vi "Plot_Rectangle.vi"(3 "Mode":T5=enum."Run VI", 5 "Traverse line In":T2={"Start X"=-1250.0, "Start Y"=-250.0, "Start Z"=180.0, "End X"=0.0, "End Y"=0.0, "End Z"=0.0, "No. of pts."=6, "Spacing"=enum."Linear", "Filename"=path "C:/Enflo_Data_Local/2015/EnFlo_Tunnel/Paul_Hayden/Calibrations/Cal_06-2015/Datum_Block_1.xls", "Tunnel Speed"=0.0, "Averaging time (min)"=0.01, "Extra Commands"="", "Carrier_1 Q (l/min)"=nan, "Carrier_2 Q (l/min)"=nan, "Trace Gas Concentration (%)"=nan, "Specific Arguments"="Datum_Image_Calibration.vi  ", "Comments"="", "Row No"=0, "Row Type Selector"=enum."Run VI Named:", "Completion time"="12:51  12-06-2015", "Row Duration (mins)"=0.11291999999999999, "No. of Valid pts."=6, "Meas Setup File"="Trav_Cam_Picture.xls"} {"Carrier_2 Q (l/min)" format="%#.2f"; "Row Duration (mins)" format="%#.1f"; "Row No" min=0; "Trace Gas Concentration (%)" min=0.0 format="%#_4f"; "Carrier_1 Q (l/min)" format="%#.2f"; "Tunnel Speed" format="%#.2f"; "Start X" format="%#.2f"; "Start Y" format="%#.2f"; "Start Z" format="%#.2f"; "End X" format="%#.2f"; "End Y" format="%#.2f"; "End Z" format="%#.2f"; "Averaging time (min)" min=0.0 format="%#.2f"}) -> (0 "Error Message":string, 1 "Status":T1, 2 "Traverse line Out":T2 {"Carrier_2 Q (l/min)" format="%#.2f"; "Row Duration (mins)" format="%#.1f"; "Row No" min=0; "Trace Gas Concentration (%)" min=0.0 format="%#_4f"; "Carrier_1 Q (l/min)" format="%#.2f"; "Tunnel Speed" format="%#.2f"; "Start X" format="%#.2f"; "Start Y" format="%#.2f"; "Start Z" format="%#.2f"; "End X" format="%#.2f"; "End Y" format="%#.2f"; "End Z" format="%#.2f"; "Averaging time (min)" min=0.0 format="%#.2f"})   [LabVIEW 2015]
uses:
  Gen Trav/Traverse_cluster.ctl
  Gen Trav/Spacing.ctl
  Controls/Multi_run_mode.ctl
  Controls/User_Specific_mode.ctl
  Gen Trav/Multi_Run_Status.ctl
panel:
  # "X           Y            Z"
  # "Start"
  # "End"
  # "X           Y            Z"
  # "Start"
  # "End"
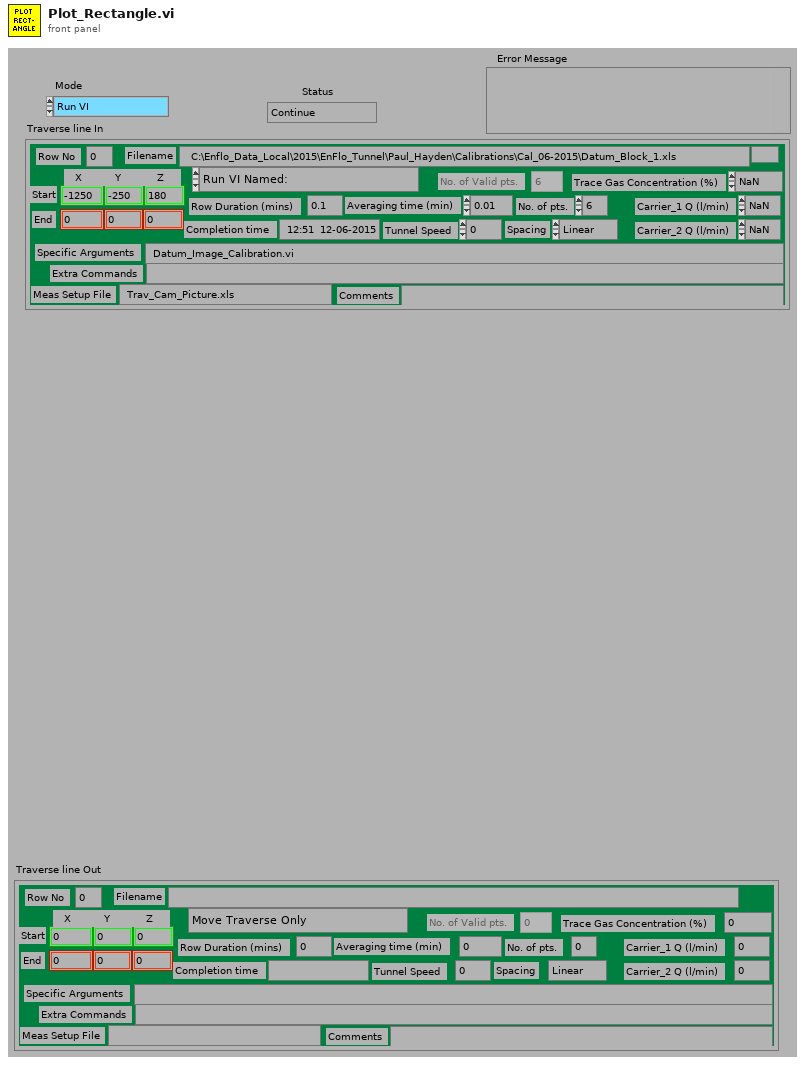
[diagram p1: front panel]
types:
  T1 = typedef "Multi_Run_Status.ctl" = enum16{"Continue", "Jump to Next Point", "Jump to Next Row", "Jump To Fall Back", "Terminate Run"}
  T2 = typedef "Traverse_cluster.ctl" = cluster{"Start X":sgl, "Start Y":sgl, "Start Z":sgl, "End X":sgl, "End Y":sgl, "End Z":sgl, "No. of pts.":i32, "Spacing":T3, "Filename":path, "Tunnel Speed":dbl, "Averaging time (min)":dbl, "Extra Commands":string, "Carrier_1 Q (l/min)":dbl, "Carrier_2 Q (l/min)":dbl, "Trace Gas Concentration (%)":dbl, "Specific Arguments":string, "Comments":string, "Row No":i32, "Row Type Selector":T4, "Completion time":string, "Row Duration (mins)":dbl, "No. of Valid pts.":i32, "Meas Setup File":string}
  T3 = typedef "Spacing.ctl" = enum16{"Linear", "Log", "Gauss", "Specified", "N/A"}
  T4 = typedef "Multi_run_mode.ctl" = enum16{"Move Traverse Only", "Set Tunnel Speed Only", "Set Source Only", "Set Measurement Conditions", "Single Measurement", "Vertical Profile", "Lateral Profile", "Longitudinal Profile", "Explore Volume", "Multi-Axis Profile", "Auto Calibrate", "Meas Fast FID Bkgnd", "Check Beam Power", "Scanning Valve Measurement", "Run VI Named:", "Set ADAM Ch", "Wait (minutes)", "Send Message", "Synchronize With:", "Fall Back to this Row", "Turn Off Row Repeating", "Blank Row", "Traverse 3D Volume"}
  T5 = typedef "User_Specific_mode.ctl" = enum16{"Check VI only", "Run VI"}
  T6 = typedef "Status_Cluster.ctl" = cluster{"Status":T1, "Error Type":string, "Error Description":string}
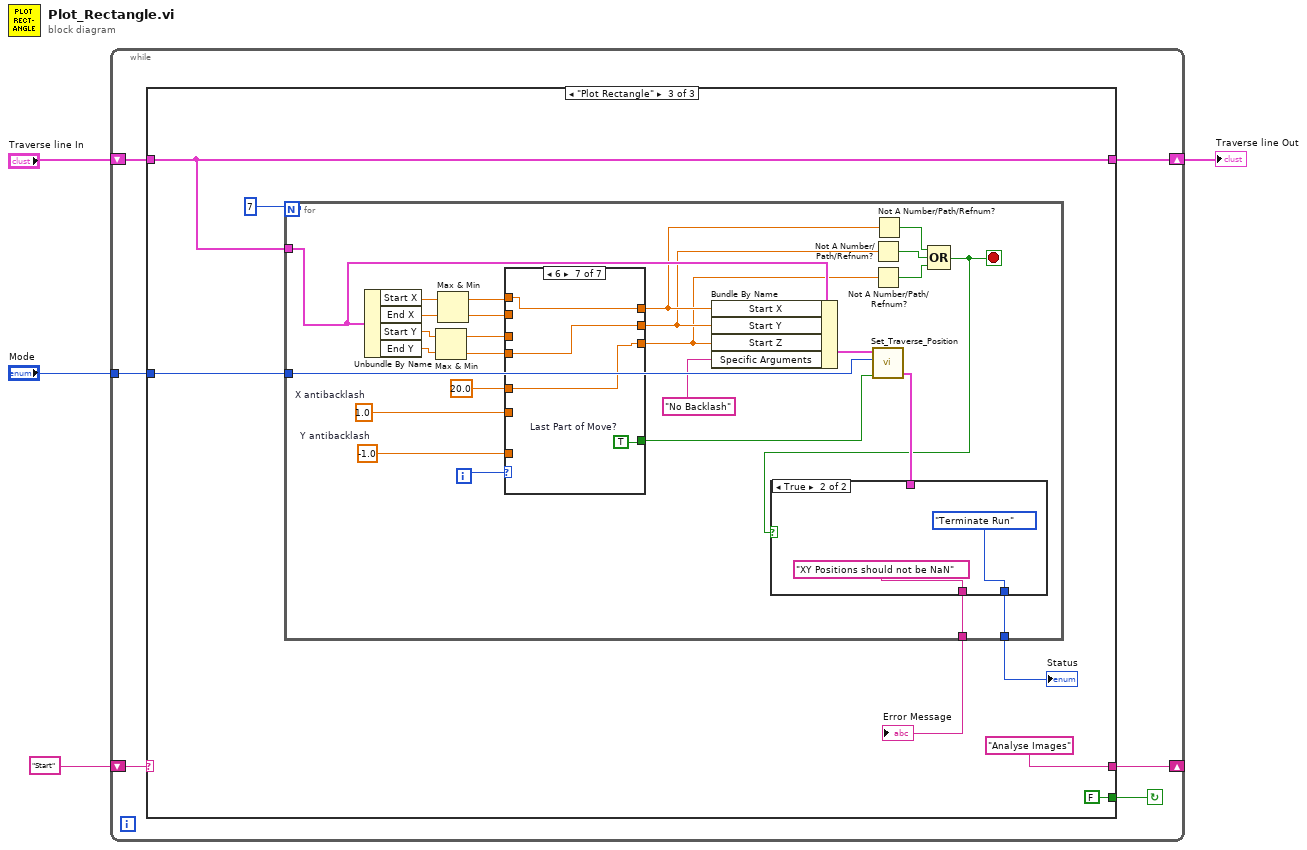
[diagram p0: block diagram]
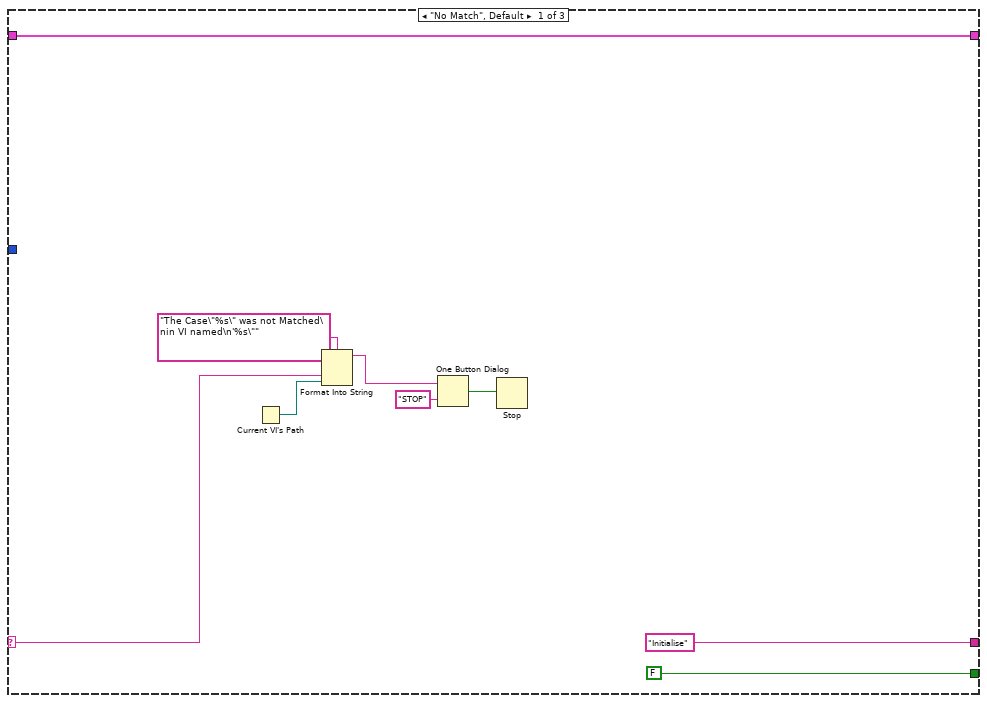
[diagram p2: hidden frame]
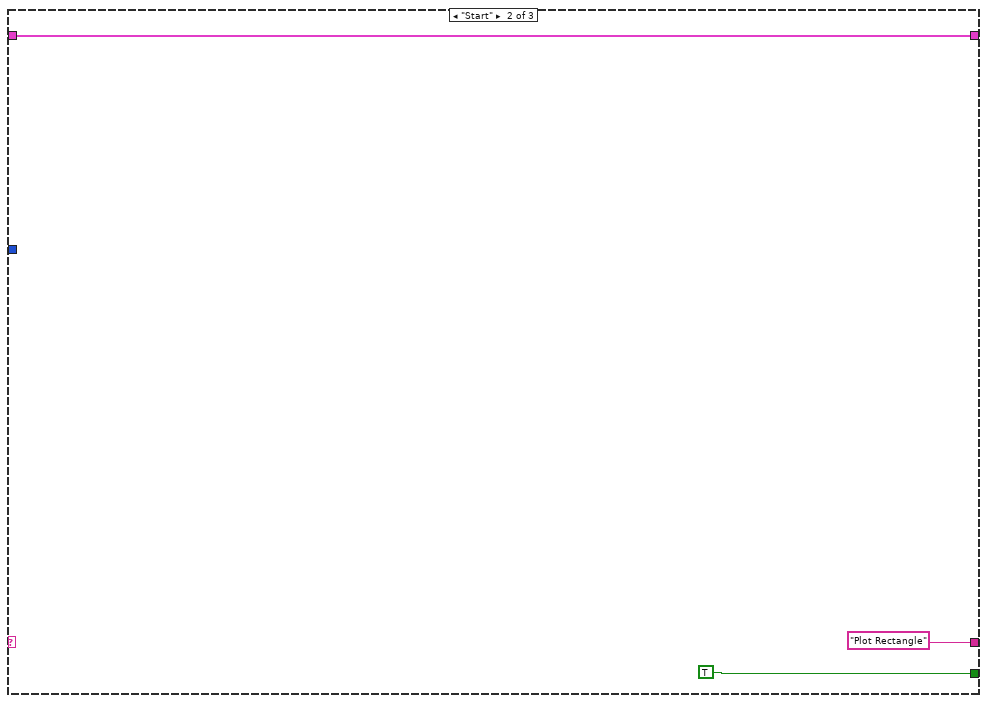
[diagram p3: hidden frame]
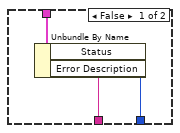
[diagram p4: hidden frame]
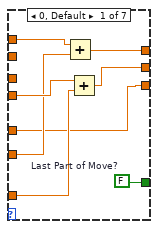
[diagram p5: hidden frame]
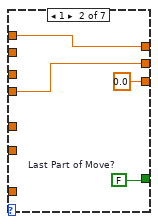
[diagram p6: hidden frame]
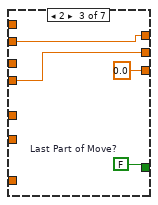
[diagram p7: hidden frame]
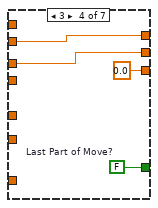
[diagram p8: hidden frame]
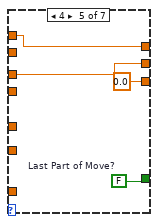
[diagram p9: hidden frame]
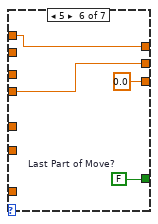
[diagram p10: hidden frame]
diagram:
  n1 = while {
    shift-left: "Start" -> [w8]
    shift-right: [w9] -> _
    tunnel: "Mode" -> [w7]
    shift-right: [w5] -> w1
    shift-left: "Traverse line In" -> [w6]
    stop <- w10 continue-if-true
    n2 = case shown="\"Plot Rectangle\"" w8 {
      selector: w8 -> [w11 _ _]
      tunnel: [FALSE TRUE FALSE] -> w10
      tunnel: ["Initialise" "Plot Rectangle" "Analyse Images"] -> w9
      tunnel: w7 -> [_ _ w27]
      tunnel: w6 -> [w12 w21 w26]
      tunnel: [w12 w21 w26] -> w5
      frame "No Match", Default {
        n3 = Current VI's Path() -> (path=w14:path)
        n4 = Format Into String(format string="The Case\"%s\" was not Matched\nin VI named\n'%s\"" ("Format String"), w11, w14) -> (resulting string=w17:string)  [unwired: 2 in, 1 out]
        n5 = One Button Dialog(message=w17, button name ("OK")="STOP") -> (true=w15:bool)
        n6 = Stop(stop? (T)=w15) -> ()
      }
      frame "Start" {
      }
      frame "Plot Rectangle" {
        n7 = for {
          N: 7 -> [_]
          tunnel: w26 -> [w56]
          tunnel: w27 -> [w55]
          tunnel: [w52] -> w24
          tunnel: [w51] -> w23
          i -> [w54]
          stop <- w31 stop-if-true
          w40 = sgl -1.0  # Y antibacklash
          w39 = sgl 1.0  # X antibacklash
          n8 = Unbundle By Name(w56) -> ("Start X"=w48:sgl, "End X"=w47:sgl, "Start Y"=w43:sgl, "End Y"=w44:sgl)
          n9 = Max & Min(x=w43, y=w44) -> (max(x,y)=w42:sgl, min(x,y)=w41:sgl)
          n10 = Max & Min(x=w48, y=w47) -> (max(x,y)=w46:sgl, min(x,y)=w45:sgl)
          n11 = case shown="6" w54 {
            tunnel: [w63 w73 w75 w79 w83 w87 w92] -> w38
            tunnel: w46 -> [w65 w73 _ _ w83 w87 w92]
            tunnel: [w66 w72 w74 w80 w82 w88 w93] -> w37
            tunnel: w41 -> [w67 w72 w74 _ _ w88 w93]
            tunnel: [w62 sgl 0.0 ("Start Y") sgl 0.0 ("Start Y") sgl 0.0 ("Start Y") sgl 0.0 ("Start Y") sgl 0.0 ("Start Y") w90] -> w36
            tunnel: w42 -> [_ _ _ w80 w82 _ _]
            tunnel: w45 -> [_ _ w75 w79 _ _ _]
            tunnel: [w69 w70 w76 w78 w84 w86 w91] -> w50
            tunnel: w40 -> [w68 _ _ _ _ _ _]
            tunnel: w39 -> [w64 _ _ _ _ _ _]
            tunnel: sgl 20.0 ("Start Y") -> [w62 _ _ _ _ _ w90]
            frame 0, Default {
              w69 = FALSE  # Last Part of Move?
              n12 = Add(x=w65, y=w64) -> (x+y=w63:sgl)
              n13 = Add(x=w67, y=w68) -> (x+y=w66:sgl)
            }
            frame 1 {
              w70 = FALSE  # Last Part of Move?
            }
            frame 2 {
              w76 = FALSE  # Last Part of Move?
            }
            frame 3 {
              w78 = FALSE  # Last Part of Move?
            }
            frame 4 {
              w84 = FALSE  # Last Part of Move?
            }
            frame 5 {
              w86 = FALSE  # Last Part of Move?
            }
            frame 6 {
              w91 = TRUE  # Last Part of Move?
            }
          }
          n14 = Bundle By Name(cluster=w56, "Start X"=w38, "Start Y"=w37, "Start Z"=w36, "Specific Arguments"="No Backlash") -> (w53:T2)
          n15 = Not A Number/Path/Refnum?(number/path/refnum=w37) -> (NaN/Path/Refnum?=w34:bool)
          n16 = Not A Number/Path/Refnum?(number/path/refnum=w36) -> (NaN/Path/Refnum?=w33:bool)
          n17 = call "Set_Traverse_Position.vi"("Last Part of Move?"=w50, "Simulate/Run"=w55, "Traverse line"=w53) -> ("Status Cluster"=w32:T6)  [unwired: 3 in]
          n18 = Not A Number/Path/Refnum?(number/path/refnum=w38) -> (NaN/Path/Refnum?=w35:bool)
          n19 = Compound Arithmetic op=OR(w35, w34, w33) -> (w31:bool)
          n20 = case shown="True" w31 {
            tunnel: w32 -> [w59 _]
            tunnel: [w58 Multi_Run_Status."Terminate Run" ("Status")] -> w52
            tunnel: [w57 "XY Positions should not be NaN" ("Error Description")] -> w51
            frame False {
              n21 = Unbundle By Name(w59) -> ("Status"=w58:T1, "Error Description"=w57:string)
            }
            frame True {
            }
          }
        }
        "Status" <- w24
        "Error Message" <- w23
      }
    }
  }
  "Traverse line Out" <- w1
